vi "Shutdown.vi"(8 "error in":errorcluster, 11 "Function Generator in":refnum<class "Function Generator.lvclass">) -> (0 "error out":errorcluster, 3 "Function Generator out":refnum<class "Function Generator.lvclass">)   [LabVIEW 2018, in "Function Generator.lvlib" / "Function Generator.lvclass"]
uses:
  Function Generator.lvclass
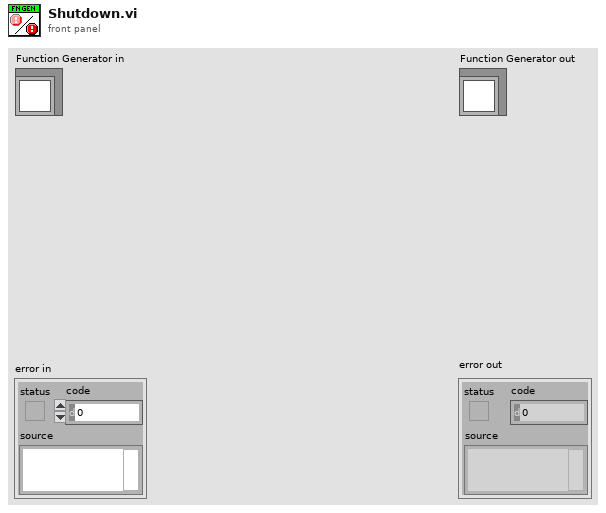
[diagram p1: front panel]
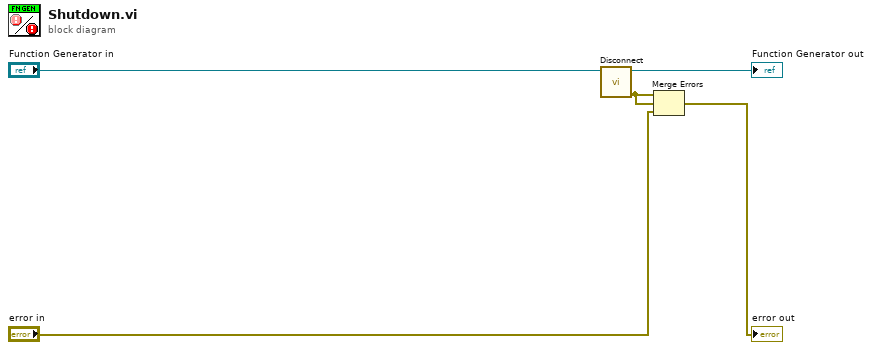
[diagram p0: block diagram]
diagram:
  n1 = call-dynamic "Disconnect.vi"("Function Generator in"="Function Generator in") -> ("error out"=w1:errorcluster, "Function Generator out"=→"Function Generator out":refnum<class "Function Generator.lvclass">)  [unwired: 9 in]
  n2 = Merge Errors(w1, w1, "error in") -> (→"error out":errorcluster)
